vi "Check SSL.vi"(9 "Input URL":string) -> (3 "Output URL":string)   [LabVIEW 2011, in "i3-twitter.lvlib"]
uses:
  i3-twitter.lvlib
  <vilib>/httpClient/LabVIEWHTTPClient.lvlib
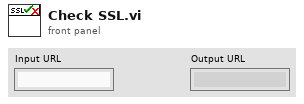
[diagram p1: front panel]
types:
  T1 = typedef "LabVIEWHTTPClient.lvlib/ClientHandle.ctl" = refnum<k1>
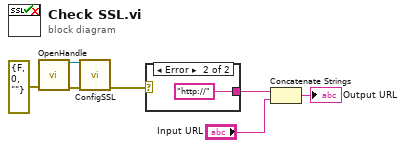
[diagram p0: block diagram]
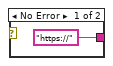
[diagram p2: hidden frame]
diagram:
  n1 = call <vilib>:"OpenHandle.vi"("error in (no error)"=errorcluster {"status"=FALSE, "code"=0, "source"=""}) -> ("client handle out"=w7:T1, "error out"=w6:errorcluster)  [unwired: 13 in]
  n2 = call <vilib>:"ConfigSSL.vi"("client handle"=w7, "error in (no error)"=w6) -> ("error out"=w5:errorcluster)  [unwired: 12 in, 1 out]
  n3 = case shown="Error" w5 {
    tunnel: ["https://" ("string") "http://" ("string")] -> w2
    frame No Error {
    }
    frame Error {
    }
  }
  n4 = Concatenate Strings(w2, "Input URL") -> (→"Output URL":string)
